vi "Sleep.vi"(8 "error in (no error)":errorcluster, 11 "Animal in":refnum<class "Animal.lvclass">) -> (0 "error out":errorcluster, 2 "Result":string, 3 "Animal out":refnum<class "Animal.lvclass">)   [LabVIEW 2020, in "Animal.lvclass"]
doc: "After sleeping animals are no longer tired. Animals cannot sleep if they are hungry."
uses:
  Animal.lvclass
  Animal.lvclass/Animal.ctl
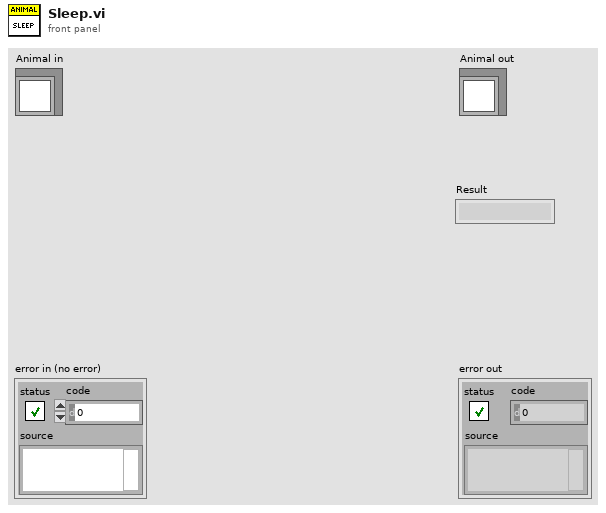
[diagram p1: front panel]
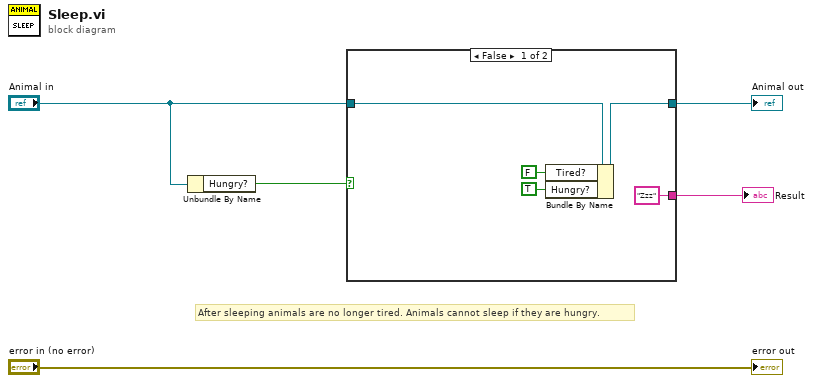
[diagram p0: block diagram]
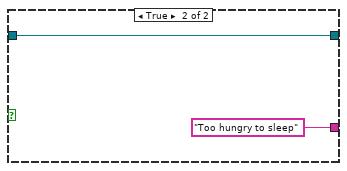
[diagram p2: hidden frame]
diagram:
  # "After sleeping animals are no longer tired. Animals cannot sleep if they are hungry."
  n1 = Unbundle By Name("Animal in") -> ("Hungry?"=w2:bool)
  n2 = case shown="False" w2 {
    tunnel: "Animal in" -> [w10 w12]
    tunnel: [w9 w12] -> w3
    tunnel: ["Zzz" "Too hungry to sleep"] -> w1
    frame False {
      n3 = Bundle By Name(cluster=w10, "Tired?"=FALSE, "Hungry?"=TRUE) -> (w9:refnum<class "Animal.lvclass">)
    }
    frame True {
    }
  }
  "Animal out" <- w3
  "Result" <- w1
  "error out" <- "error in (no error)"
